vi "Set LTS Stage Enabled.vi"(8 "error in (no error)":errorcluster, 10 "Cluster in":T1, 11 "LTS Reference In":refnum<k24>) -> (0 "error out":errorcluster, 2 "Cluster out":T1, 3 "LTS Reference Out":refnum<k24>)   [LabVIEW 2014]
uses:
  Ctrls/Translation Stage Cluster.ctl
  C:/Projects/Serial Sectioning OCT - TortoiseGIT/SerialSectOCT/Software/Test Code/Thorlabs.MotionControl.Controls.dll
  Thorlabs.MotionControl.Controls.dll
  C:/Projects/Serial Sectioning OCT - TortoiseGIT/SerialSectOCT/Software/Thorlabs.MotionControl.IntegratedStepperMotorsCLI.dll
  Thorlabs.MotionControl.IntegratedStepperMotorsCLI.dll
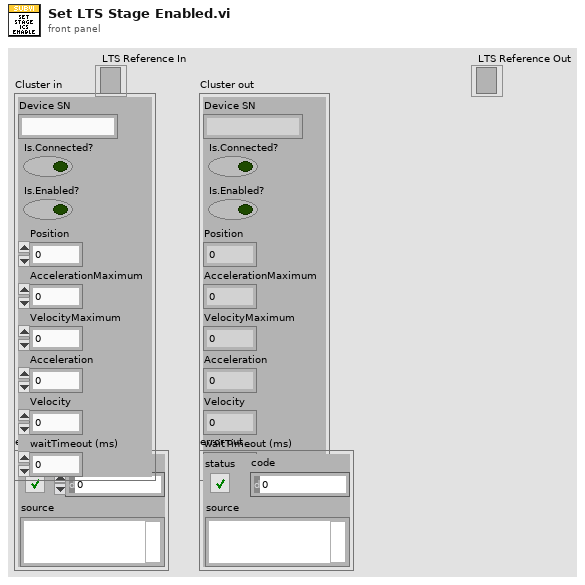
[diagram p1: front panel]
types:
  T1 = typedef "Translation Stage Cluster.ctl" = cluster{"Device SN":string, "Is.Connected?":bool, "Is.Enabled?":bool, "Position":dbl, "AccelerationMaximum":dbl, "VelocityMaximum":dbl, "Acceleration":dbl, "Velocity":dbl, "waitTimeout (ms)":i32}
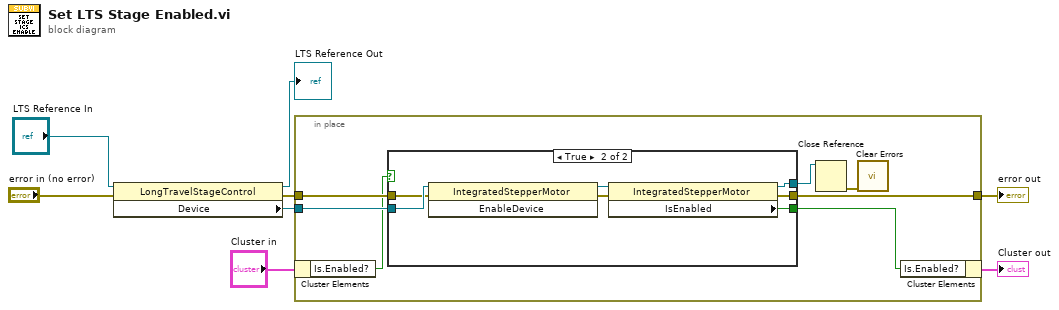
[diagram p0: block diagram]
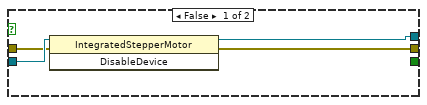
[diagram p2: hidden frame]
diagram:
  n1 = property class="LongTravelStageControl"(reference="LTS Reference In", error in="error in (no error)") -> (reference out=→"LTS Reference Out":refnum<k24>, error out=w6:errorcluster, "Device"=w2:refnum<k24>)
  n2 = in-place {
    in-place-border: w2 -> [w15]
    in-place-border: w6 -> [w14]
    in-place-border: [w13] -> w4
    n3 = in-place-cluster #1("Cluster in") -> ("Is.Enabled?"=w9:bool)
    n4 = case shown="True" w9 {
      tunnel: w15 -> [w19 w26]
      tunnel: w14 -> [w18 w25]
      tunnel: [w17 w23] -> w13
      tunnel: [w16 w21] -> w11
      tunnel: [_ w20] -> w10
      frame False {
        n5 = invoke class="IntegratedStepperMotor" method="DisableDevice"(reference=w19, error in=w18) -> (reference out=w16:refnum<k24>, error out=w17:errorcluster)  [unwired: 1 in, 1 out]
      }
      frame True {
        n6 = invoke class="IntegratedStepperMotor" method="EnableDevice"(reference=w26, error in=w25) -> (reference out=w22:refnum<k24>, error out=w24:errorcluster)  [unwired: 1 in, 1 out]
        n7 = property class="IntegratedStepperMotor"(reference=w22, error in=w24) -> (reference out=w21:refnum<k24>, error out=w23:errorcluster, "IsEnabled"=w20:bool)
      }
    }
    n8 = Close Reference(reference=w11) -> (error out=w12:errorcluster)  [unwired: 1 in]
    n9 = call <vilib>:"Clear Errors.vi"("error in (no error)"=w12) -> ()  [unwired: 5 in, 2 out]
    n10 = in-place-cluster #1("Is.Enabled?"=w10) -> (→"Cluster out":T1)
  }
  "error out" <- w4
